vi "DeadbandCounter.vi"(0 "Input":bool, 1 "Enable":bool, 2 "Deadtime":u16=1, 11 "stateIn":u16=1) -> (4 "Output":bool, 15 "stateOut":u16)   [LabVIEW 2017, in "BuckBoost.lvlib"]
uses:
  BuckBoost.lvlib
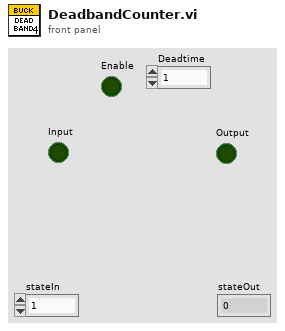
[diagram p1: front panel]
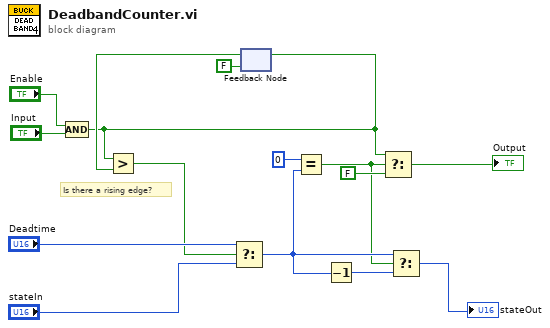
[diagram p0: block diagram]
diagram:
  # "Is there a rising edge?"
  n1 = Compound Arithmetic op=AND("Enable", "Input") -> (w7:bool)
  n2 = feedback #1(FALSE) -> (w11:bool)
  n3 = Greater?(x=w7, y=w11) -> (0:w2:bool)
  n4 = Select(t="Deadtime", s=w2, f="stateIn") -> (s? t:f=w5:u16)
  n5 = feedback-in #1(w7) -> ()
  n6 = Equal?(x=u16 0, y=w5) -> (x = y?=w3:bool)
  n7 = Decrement(x=w5) -> (x-1=w6:u16)
  n8 = Select(t=w7, s=w3, f=FALSE) -> (s? t:f=→"Output":bool)
  n9 = Select(t=w5, s=w3, f=w6) -> (s? t:f=→"stateOut":u16)
